vi "nufern common operation test.vi"() -> ()   [LabVIEW 2016]
uses:
  Common Operation Control 1.ctl
  Logistics Control 2.ctl
  2 digit hex indicator.ctl
  Extended Operation Control 3.ctl
  sniper current tests/Return Code Cluster.ctl
  producer enum control.ctl
  sniper current tests/Unit Status Cluster Control 1.ctl
  sniper current tests/Status  Cluster.ctl
  sniper current tests/Fault Cluster.ctl
  <vilib>/Instr/_visa.llb/VISA Configure Serial Port (Instr).vi
  <extravilib>/ChannelInstances/One Element Stream-i32/Instantiate.vi
  <extravilib>/ChannelInstances/One Element Stream-i32/EndpointRead.vi
  <extravilib>/ChannelInstances/One Element Stream-i32/Endpoint.vi
  <extravilib>/ChannelInstances/One Element Stream-i32.lvlib
panel:
  out "Fault Cluster":T1
  out "Status Cluster":T2
  out "inside Common Operation":bool
  out "Unit Status Cluster":T3={"laser serial number"=0, "Firmware Part Number"=0, "Firmware Version Major"=1, "Firmware Version Minor"=1, "Firmware Version Bugfix"=1, "Gateware Part Number"=0, "Gateware Version Minor"=1, "Gateware Version Major"=1, "Gateware Version Bugfix"=1, "Valid Readings"=FALSE} {"Gateware Version Bugfix" format="0x%02x"; "Gateware Version Major" format="0x%02x"; "Gateware Version Minor" format="0x%02x"; "Gateware Part Number" format="0x%04x"; "Firmware Version Bugfix" format="0x%02x"; "Firmware Version Minor" format="0x%02x"; "Firmware Version Major" format="0x%02x"; "Firmware Part Number" format="0x%04x"}
  out "return count 2":u32
  out "read buffer":string
  in  "control":T5=enum."Common Operation"
  out "New Value Could not be parsed":bool
  out "New value is outside \nof the inclusive range of 1-99%":bool
  out "Fault Status Cluster":T6
  out "Extended Status Cluster":T7 {"Temperature Array" format="0x%02x"; "Back-Reflection" format="0x%08x"; "HPE Threshold" format="0x%08x"; "HPE Monitor" format="0x%08x"; "Stage 2 Output Monitor" format="0x%08x"; "Stage 1 Input Monitor" format="0x%08x"; "Stage 2 Current" format="0x%08x"; "Stage 1 Current" format="0x%08x"; "Extended Status Return Code" format="0x%02x"}
  out "Back-Reflection Reading":u32 format="0x%08x"
  out "Return Code Cluster":T8 {"Current RS-485 \nAddress" format="0x%02x"; "Desired RS-485 \nAddress" format="0x%02x"; "Set Power Mode Return Code" format="0x%02x"; "Clear Faults Return Code" format="0x%02x"; "Return Code Description" items=["Accepted/No Error", "Incorrect Message Format", "Incorrect Message Length", "CRC Error", "Unrecognized Command", "Argument Out of Range", "Argument Parse Error", "Operation Not Permitted", "Operation Failed"]; "Get RS-485 Address \nReturn Code" format="0x%02x"; "Set RS-485 Address \nReturn Code" format="0x%02x"; "Set Power Mode Return Code" format="0x%02x"; "Clear Faults Return Code" format="0x%02x"; "Extended Status Return Code" format="0x%02x"}
  out "HPE Photodiode Reading":u32 format="0x%08x"
  out "Laser is in High Power Mode":bool
  out "aborted?":bool
  in  "timeout (s)":dbl=1.0 format="%#_13g"
  out "consumer loop":i32
  out "stop consumer":bool
  out "producer loop":i32
  out "stop producer":bool
  in  "stop":bool
  out "return count":u32
  out "string out to nufern":string
  in  "PAPA Address":i8=1 format="0x%02x"
  in  "Calibration":T9 {"Common Operation" format="0x%d" items=["Undefined", "Query: Get Unit Information", "Cmd: Emission On", "Cmd: Emission Off", "Query: Get Basic Status", "Query: Get Core Status", "Query: Get Extended Status", "Cmd: Clear Faults", "Cmd: Set Power Mode"]}
  in  "Extended Operation":T10={"Extended Operation"=0, "OK Button"=FALSE, " HPE Photodiode \nSignal Drop Tolerance"=0.99} {"HPE Photodiode \nSignal Drop Tolerance" min=0.01 max=0.99 step=0.01 format="%#_g%%"; "Extended Operation" format="0x%x" items=["undefined"=0, "Set HPE Photodiode Signal Drop Tolerance"=67, "Get HPE Photodiode Signal Drop Tolerance"=68, "Switch HPE Photodiode Fault Enable"=69, "Get Temperature Sensor Status"=70, "Switch Communication Timeout Enable"=71]}
  in  "Logistics":T11={"Logistics"=66, "OK Button"=FALSE, "Desired RS-485 \nAddress "=0, "Current RS-485 \nAddress "=0} {"Current RS-485 \nAddress" format="0x%02x"; "Desired RS-485 \nAddress" format="0x%02x"; "Logistics" format="0x%x" items=["Set RS-485 Address"=65, "Get RS-485 Address"=66]}
  in  "Common Operation":T9={"Common Operation"=1, "OK Button"=FALSE} {"Common Operation" format="0x%d" items=["Undefined", "Query: Get Unit Information", "Cmd: Emission On", "Cmd: Emission Off", "Query: Get Basic Status", "Query: Get Core Status", "Query: Get Extended Status", "Cmd: Clear Faults", "Cmd: Set Power Mode"]}
  out "error out":errorcluster
  in  "error in (no error)":errorcluster
  in  "baud rate (9600)":u32=115200
  in  "VISA resource name":refnum<visa-resource-name>="COM1"
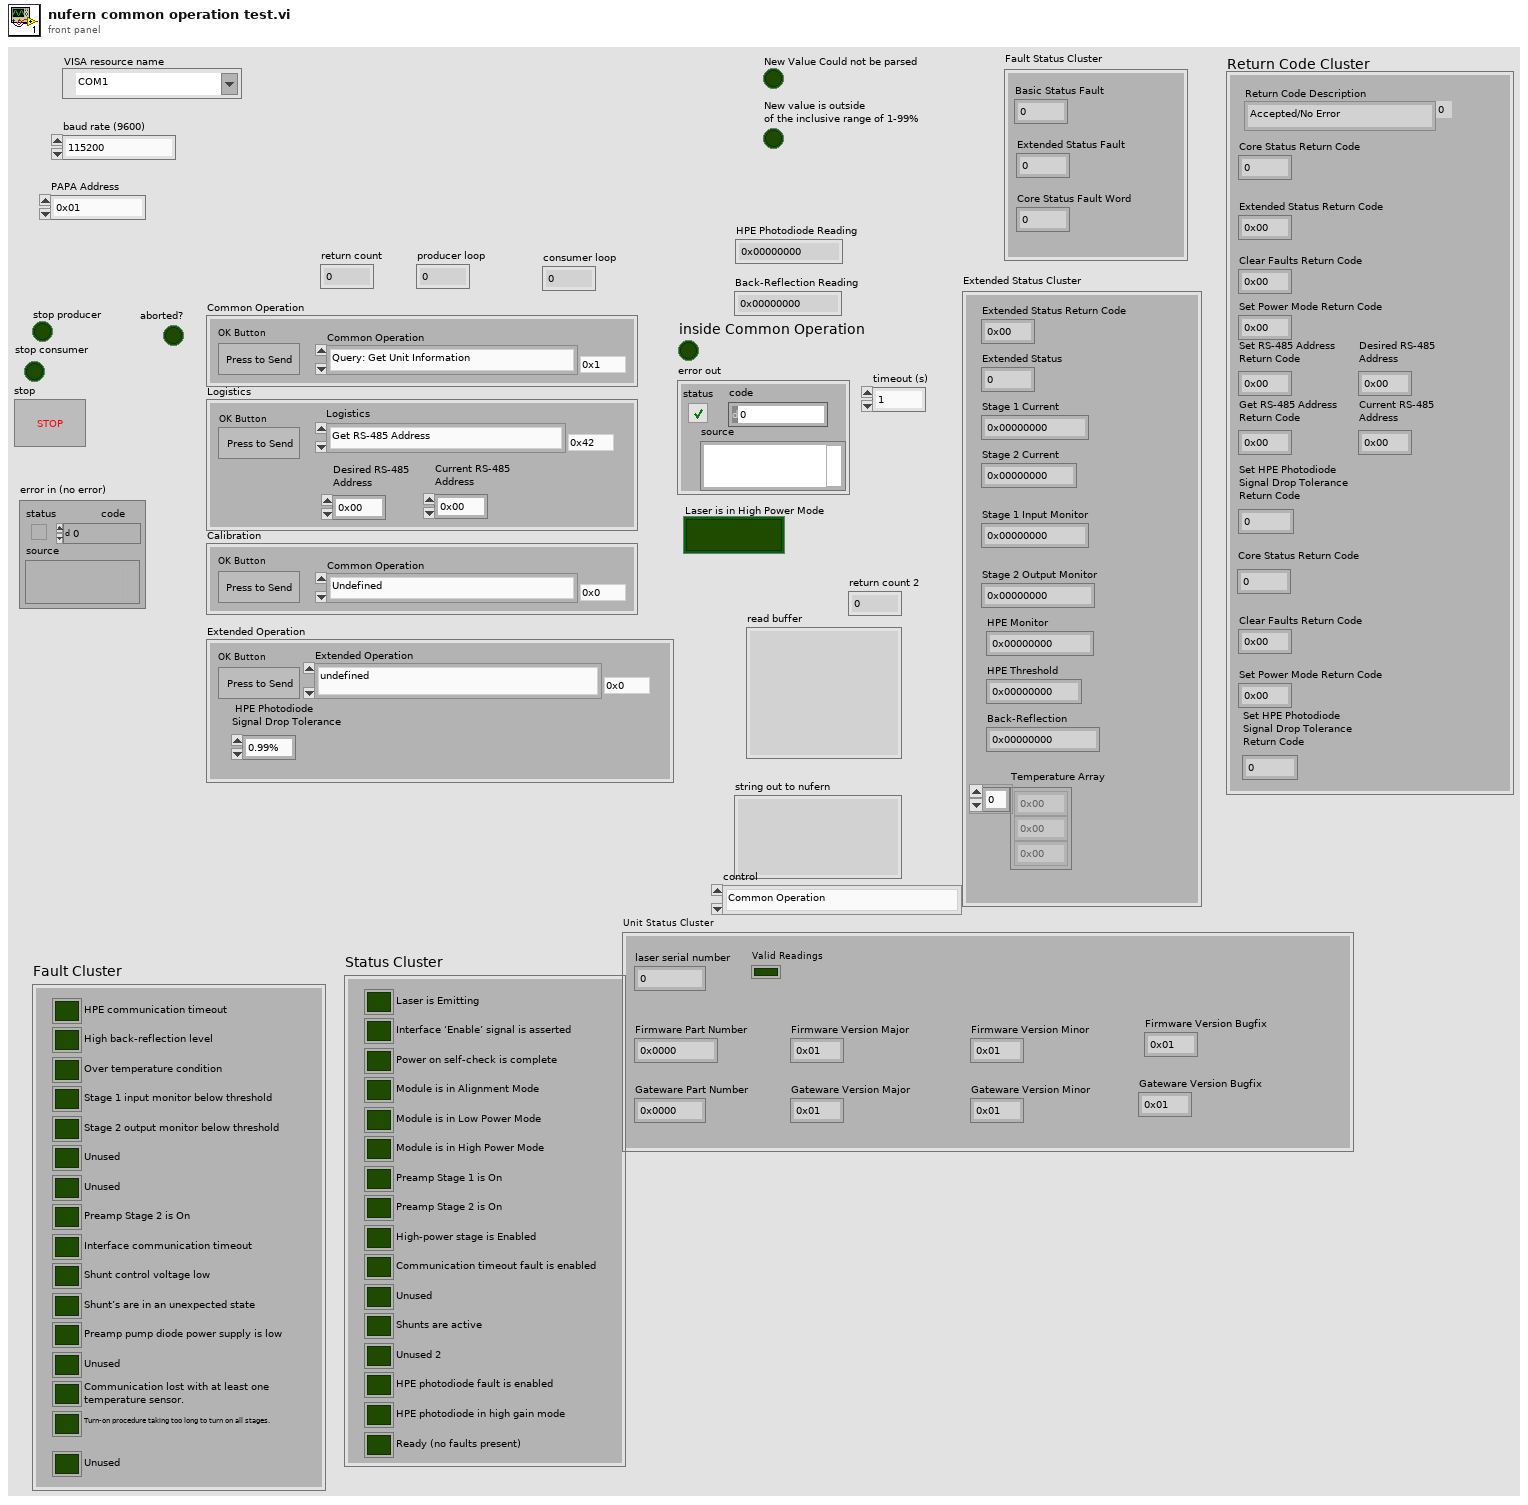
[diagram p1: front panel]
types:
  T1 = typedef "Fault Cluster.ctl" = cluster{"HPE communication timeout":bool, "High back-reflection level":bool, "Over temperature condition":bool, "Stage 1 input monitor below threshold":bool, "Stage 2 output monitor below threshold":bool, "Unused":bool, "Unused":bool, "Preamp Stage 2 is On":bool, "Interface communication timeout":bool, "Shunt control voltage low":bool, "Shunt’s are in an unexpected state":bool, "Preamp pump diode power supply is low":bool, "Unused":bool, "Communication lost with at least one\ntemperature sensor.":bool, "Turn-on procedure taking too long to turn on all stages.":bool, "Unused":bool}
  T2 = typedef "Status  Cluster.ctl" = cluster{"Laser is Emitting":bool, "Interface ‘Enable’ signal is asserted":bool, "Power on self-check is complete":bool, "Module is in Alignment Mode":bool, "Module is in Low Power Mode":bool, "Module is in High Power Mode":bool, "Preamp Stage 1 is On":bool, "Preamp Stage 2 is On":bool, "High-power stage is Enabled":bool, "Communication timeout fault is enabled":bool, "Unused":bool, "Shunts are active":bool, "Unused 2":bool, "HPE photodiode fault is enabled":bool, "HPE photodiode in high gain mode":bool, "Ready (no faults present)":bool}
  T3 = typedef "Unit Status Cluster Control 1.ctl" = cluster{"laser serial number":u32, "Firmware Part Number":u32, "Firmware Version Major":T4, "Firmware Version Minor":T4, "Firmware Version Bugfix":T4, "Gateware Part Number":u32, "Gateware Version Minor":T4, "Gateware Version Major":T4, "Gateware Version Bugfix":T4, "Valid Readings":bool}
  T4 = typedef "2 digit hex indicator.ctl" = i32
  T5 = typedef "producer enum control.ctl" = enum16{"Timeout", "Stop", "Common Operation", "Calibration", "Extended Operation", "Logistics"}
  T6 = cluster{"Basic Status Fault":u32, "Core Status Fault Word":u32, "Extended Status Fault":u32}
  T7 = cluster{"Extended Status Return Code":T4, "Extended Status ":u32, "Stage 1 Current":u32, "Stage 2 Current":u32, "Stage 1 Input Monitor":u32, "Stage 2 Output Monitor":u32, "HPE Monitor":u32, "HPE Threshold":u32, "Back-Reflection":u32, "Temperature Array":T4[]}
  T8 = typedef "Return Code Cluster.ctl" = cluster{"Core Status Return Code":u32, "Extended Status Return Code":T4, "Clear Faults Return Code":T4, "Set Power Mode Return Code":T4, "Set RS-485 Address \nReturn Code":T4, "Get RS-485 Address \nReturn Code":T4, "Set HPE Photodiode \nSignal Drop Tolerance \nReturn Code":u32, "Return Code Description":u16, "Core Status Return Code":u32, "Clear Faults Return Code":T4, "Set Power Mode Return Code ":T4, "Desired RS-485 \nAddress ":T4, "Current RS-485 \nAddress ":T4, "Set HPE Photodiode \nSignal Drop Tolerance \nReturn Code ":u32}
  T9 = typedef "Common Operation Control 1.ctl" = cluster{"Common Operation":u16, "OK Button":bool}
  T10 = typedef "Extended Operation Control 3.ctl" = cluster{"Extended Operation":u16, "OK Button":bool, " HPE Photodiode \nSignal Drop Tolerance":dbl}
  T11 = typedef "Logistics Control 2.ctl" = cluster{"Logistics":u16, "OK Button":bool, "Desired RS-485 \nAddress ":T4, "Current RS-485 \nAddress ":T4}
  T12 = typedef "One Element Stream-i32.lvlib/)Channel.ctl" = refnum<queue>
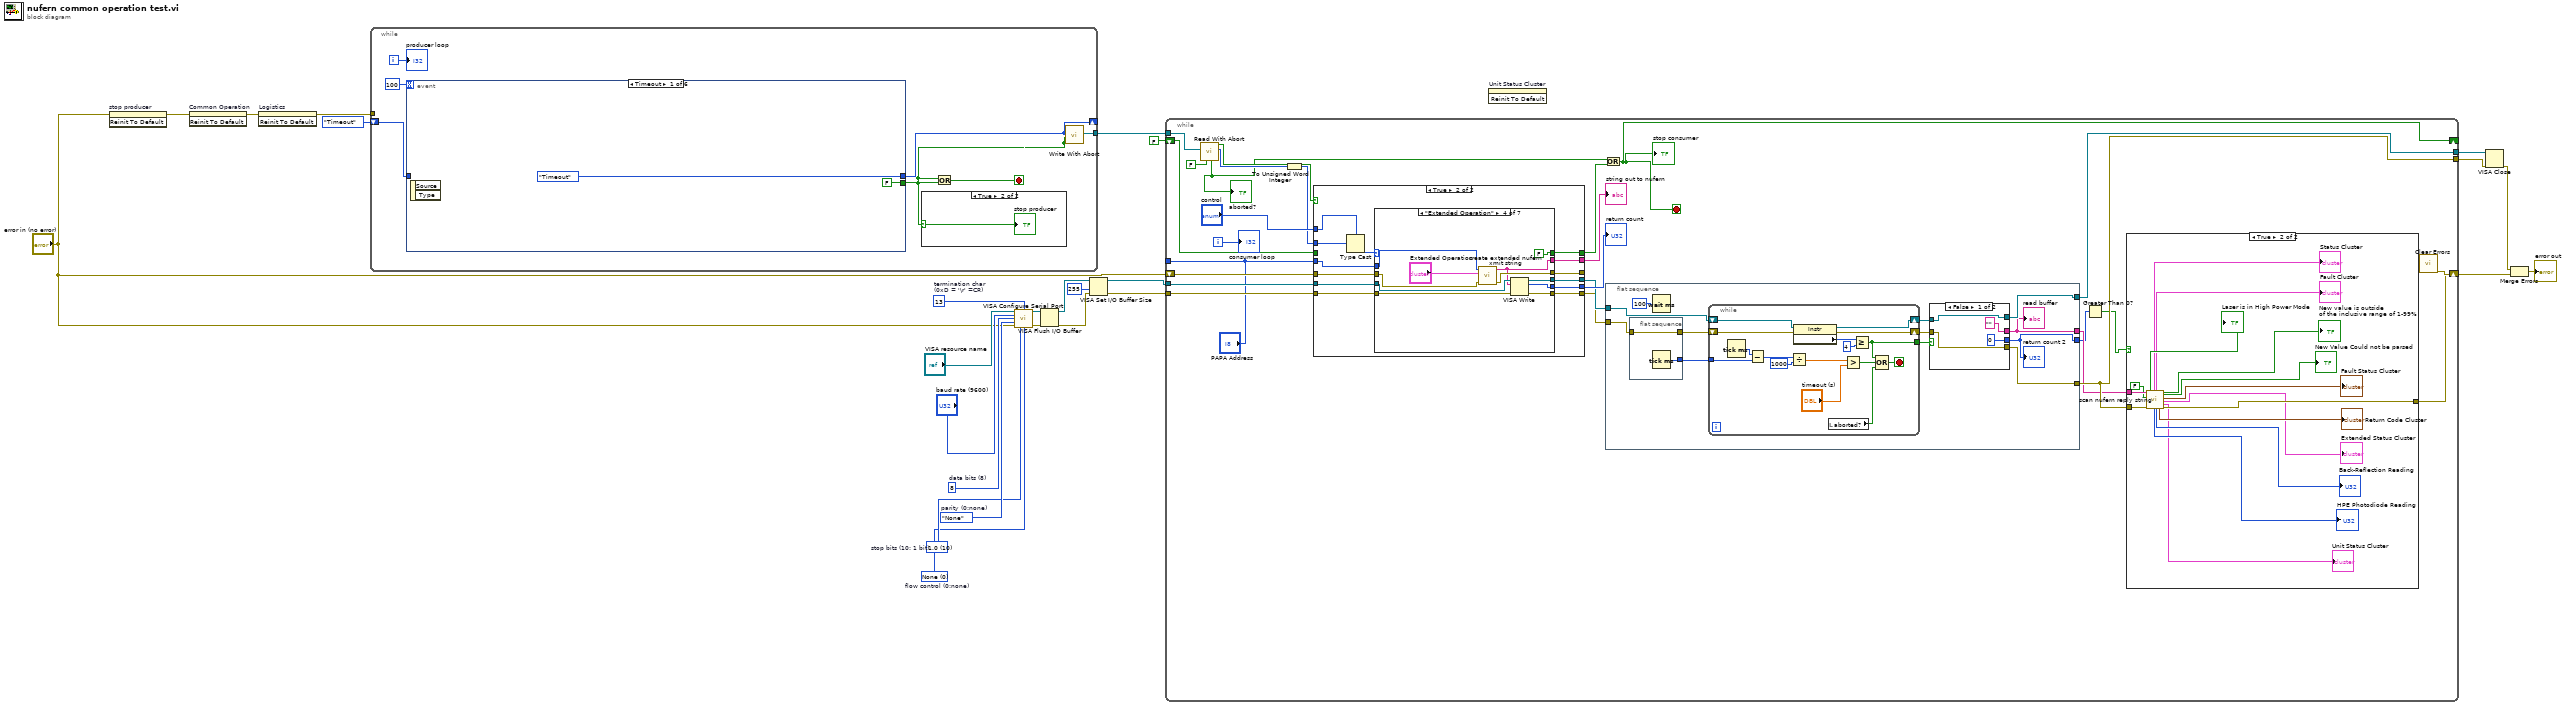
[diagram p0: block diagram]
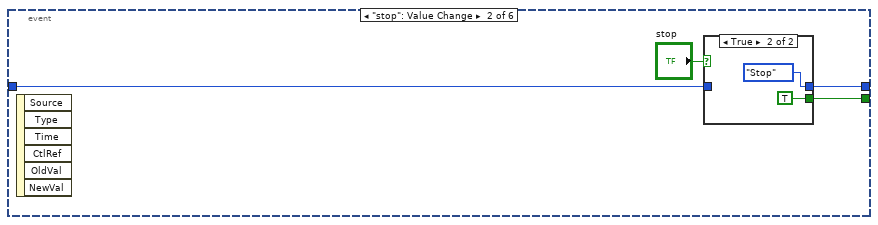
[diagram p2: hidden frame]
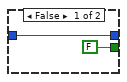
[diagram p3: hidden frame]
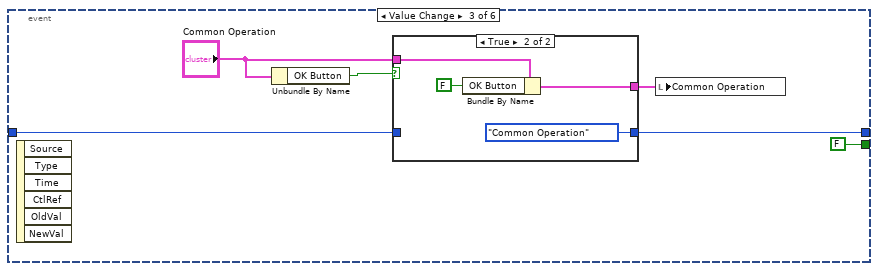
[diagram p4: hidden frame]
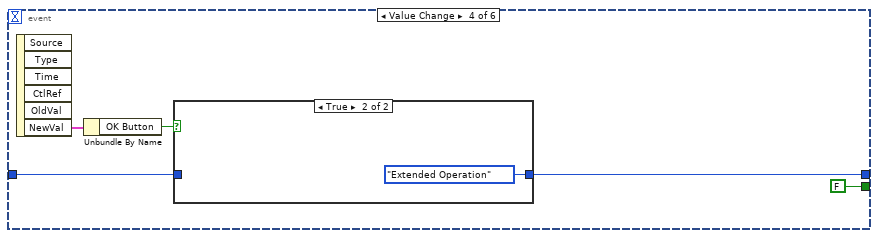
[diagram p6: hidden frame]
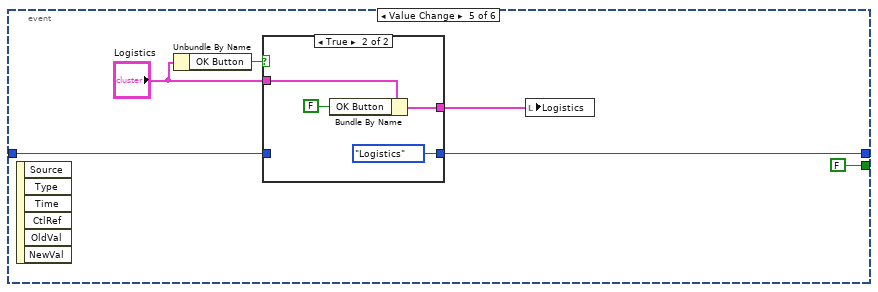
[diagram p8: hidden frame]
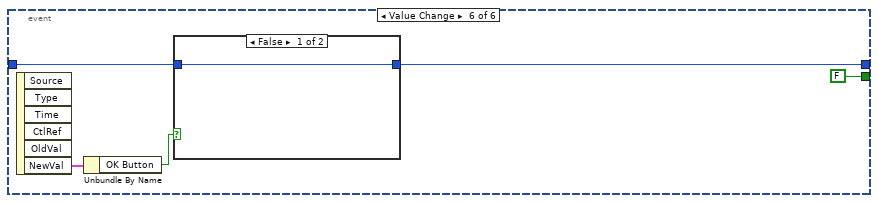
[diagram p10: hidden frame]
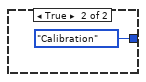
[diagram p11: hidden frame]
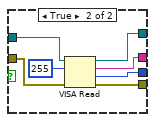
[diagram p14: hidden frame]
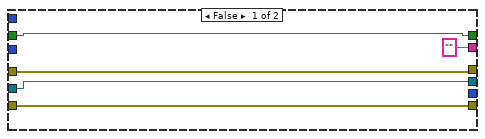
[diagram p15: hidden frame]
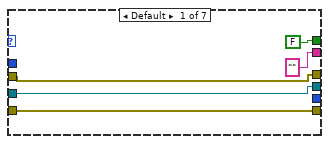
[diagram p16: hidden frame]
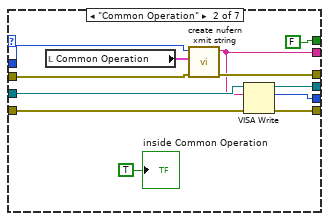
[diagram p17: hidden frame]
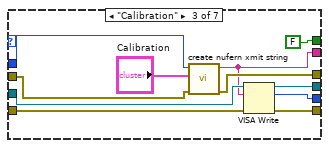
[diagram p18: hidden frame]
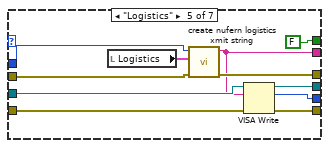
[diagram p19: hidden frame]
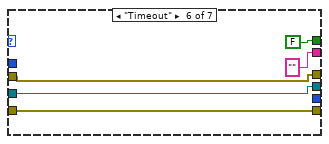
[diagram p20: hidden frame]
diagram:
  w18 = u8 13  # termination char (0xD = '\r' =CR)
  w21 = u16 0 items=["None", "XON/XOFF", "RTS/CTS", "XON/XOFF & RTS/CTS", "DTR/DSR", "XON/XOFF & DTR/DSR"]  # flow control (0:none)
  w22 = u16 10 items=["1.0"=10, "1.5"=15, "2.0"=20]  # stop bits (10: 1 bit)
  w23 = enum16{"None", "Odd", "Even", "Mark", "Space"}."None"  # parity (0:none)
  w24 = u16 8  # data bits (8)
  n1 = invoke on="stop producer" class="Bool (strict)" method="Reinit To Default"(error in="error in (no error)") -> (error out=w1:errorcluster)  [unwired: 2 in, 2 out]
  n2 = invoke on="Common Operation" class="Clust (strict)" method="Reinit To Default"(error in=w1) -> (error out=w4:errorcluster)  [unwired: 2 in, 2 out]
  n3 = invoke on="Logistics" class="Clust (strict)" method="Reinit To Default"(error in=w4) -> (error out=w3:errorcluster)  [unwired: 2 in, 2 out]
  n4 = while {
    tunnel: [w31] -> w12
    shift-right: [w28] -> _
    shift-left: producer_enum_control."Timeout" -> [w29]
    tunnel: w3 -> [_]
    i -> [w32]
    stop <- w30 stop-if-true
    n5 = event shown="[0] Timeout" {
      selector: _ -> [_ _ _ _ _ _]
      dyn-events: _ -> [_ _ _ _ _ _]
      timeout: 100 -> [_ _ _ _ _ _]
      tunnel: [producer_enum_control."Timeout" w38 w49 w60 w68 w79] -> w28
      tunnel: w29 -> [_ w36 w47 w57 w66 w76]
      tunnel: [FALSE w37 FALSE FALSE FALSE FALSE] -> w27
      event Timeout {
        n6 = event-data() -> ()  [unwired: 1 in, 2 out]
      }
      event "stop": Value Change {
        n7 = event-data() -> ()  [unwired: 1 in, 6 out]
        n8 = case shown="True" "stop" {
          tunnel: [w40 producer_enum_control."Stop"] -> w38
          tunnel: [FALSE TRUE] -> w37
          tunnel: w36 -> [w40 _]
          frame False {
          }
          frame True {
          }
        }
      }
      event Value Change {
        n9 = event-data() -> ()  [unwired: 1 in, 6 out]
        n10 = Unbundle By Name("Common Operation") -> ("OK Button"=w46:bool)
        n11 = case shown="True" w46 {
          tunnel: [w51 producer_enum_control."Common Operation"] -> w49
          tunnel: w47 -> [w51 _]
          tunnel: [w50 w53] -> w45
          tunnel: "Common Operation" -> [w50 w54]
          frame False {
          }
          frame True {
            n12 = Bundle By Name(cluster=w54, "OK Button"=FALSE) -> (w53:T9)
          }
        }
        n13 = local write "Common Operation"(w45) -> ()
      }
      event Value Change {
        n14 = event-data() -> ("NewVal"=w58:T10)  [unwired: 1 in, 5 out]
        n15 = Unbundle By Name(w58) -> ("OK Button"=w56:bool)
        n16 = case shown="True" w56 {
          tunnel: [w61 producer_enum_control."Extended Operation"] -> w60
          tunnel: w57 -> [w61 _]
          frame False {
          }
          frame True {
          }
        }
      }
      event Value Change {
        n17 = event-data() -> ()  [unwired: 1 in, 6 out]
        n18 = Unbundle By Name("Logistics") -> ("OK Button"=w65:bool)
        n19 = case shown="True" w65 {
          tunnel: [w70 producer_enum_control."Logistics"] -> w68
          tunnel: w66 -> [w70 _]
          tunnel: [w69 w72] -> w64
          tunnel: "Logistics" -> [w69 w73]
          frame False {
          }
          frame True {
            n20 = Bundle By Name(cluster=w73, "OK Button"=FALSE) -> (w72:T11)
          }
        }
        n21 = local write "Logistics"(w64) -> ()
      }
      event Value Change {
        n22 = event-data() -> ("NewVal"=w77:T9)  [unwired: 1 in, 5 out]
        n23 = Unbundle By Name(w77) -> ("OK Button"=w75:bool)
        n24 = case shown="False" w75 {
          tunnel: [w80 producer_enum_control."Calibration"] -> w79
          tunnel: w76 -> [w80 _]
          frame False {
          }
          frame True {
          }
        }
      }
    }
    n25 = case shown="True" w27 {
      selector: w27 -> [_ w82]
      frame False {
      }
      frame True {
        "stop producer" <- w82
      }
    }
    n26 = Or(x=w27, y=w27) -> (x .or. y?=w30:bool)
    n27 = call <extravilib>:"Write With Abort.vi"("abort"=w27, "last element? (F)"=w27, "element"=w28) -> ("channel"=w31:T12)  [unwired: 6 in, 2 out]
    "producer loop" <- w32
  }
  n28 = call-poly "VISA Configure Serial Port"("VISA resource name"="VISA resource name", "termination char\n(0xA = '\\n' = LF)"=w18, "baud rate (9600)"="baud rate (9600)", "data bits (8)"=w24, "parity (0:none)"=w23, "error in (no error)"="error in (no error)", "stop bits (10: 1 bit)"=w22, "flow control (0:none)"=w21) -> ("VISA resource name out"=w19:refnum<visa-resource-name>, "error out"=w20:errorcluster)  [unwired: 6 in]
  n29 = VISA Flush I/O Buffer(VISA resource name=w19, error in (no error)=w20) -> (VISA resource name out=w15:refnum<visa-resource-name>, error out=w7:errorcluster)  [unwired: 1 in]
  n30 = VISA Set I/O Buffer Size(VISA resource name=w15, size (4096)=u32 255, error in (no error)=w7) -> (VISA resource name out=w8:refnum<visa-resource-name>, error out=w6:errorcluster)  [unwired: 1 in]
  n31 = while {
    shift-right: [w93] -> w9
    shift-left: "error in (no error)" -> [w108]
    tunnel: w8 -> [w107]
    tunnel: [w91] -> w14
    tunnel: w6 -> [w106]
    tunnel: [w90] -> w13
    tunnel: ["PAPA Address"] -> _
    tunnel: w12 -> [w104]
    shift-right: [w95] -> _
    shift-left: FALSE -> [w98]
    i -> [w100]
    stop <- w95 stop-if-true
    n32 = call <extravilib>:"Read With Abort.vi"("abort"=FALSE, "channel"=w104) -> ("element"=w102:i32, "element valid?"=w103:bool, "aborted?"=w94:bool)  [unwired: 5 in, 2 out]
    "aborted?" <- w94
    n33 = To Unsigned Word Integer(number=w102) -> (unsigned 16bit integer=w85:u16)
    n34 = case shown="True" w103 {
      tunnel: [w168 w183] -> _
      tunnel: w108 -> [w168 w182]
      tunnel: w107 -> [w170 w181]
      tunnel: "PAPA Address" -> [_ w180]
      tunnel: [w170 w179] -> w97
      tunnel: w106 -> [w169 w178]
      tunnel: [w169 w177] -> w96
      tunnel: ["" ("String Out to nufern") w176] -> w89
      tunnel: [_ w175] -> w105
      tunnel: "control" -> [_ w173]
      tunnel: w85 -> [_ w171]
      tunnel: [w166 w174] -> w99
      tunnel: w98 -> [w166 _]
      frame False {
      }
      frame True {
        n35 = Type Cast(type=w173, x=w171) -> (*(type *) &x=w172:T5)
        n36 = case shown="\"Extended Operation\"" w172 {
          tunnel: [w186 w200 w211 w222 w233 w237 w241] -> w183
          tunnel: w182 -> [w186 w199 w210 w221 w232 w237 w241]
          tunnel: w181 -> [w188 w198 w209 w220 w231 w235 w239]
          tunnel: w180 -> [_ w197 w208 w219 w230 _ _]
          tunnel: [w188 w196 w207 w218 w229 w235 w239] -> w179
          tunnel: w178 -> [w187 w195 w206 w217 w228 w236 w240]
          tunnel: [w187 w194 w205 w216 w227 w236 w240] -> w177
          tunnel: ["" ("String Out to nufern") w191 w204 w215 w226 "" ("String Out to nufern") _] -> w176
          tunnel: [_ w193 w203 w214 w225 _ _] -> w175
          tunnel: [FALSE FALSE FALSE FALSE FALSE FALSE TRUE] -> w174
          frame Default {
          }
          frame "Common Operation" {
            n37 = local read "Common Operation"() -> (w190:T9)
            n38 = call "create nufern xmit string.vi"("error in (no error)"=w199, "Common Operation"=w190, "PAPA Address"=w197) -> ("error out"=w200:errorcluster, "String Out to nufern"=w191:string)  [unwired: 5 in, 2 out]
            n39 = VISA Write(VISA resource name=w198, write buffer=w191, error in (no error)=w195) -> (VISA resource name out=w196:refnum<visa-resource-name>, return count=w193:u32, error out=w194:errorcluster)
            "inside Common Operation" <- TRUE
          }
          frame "Calibration" {
            n40 = call "create nufern xmit string.vi"("error in (no error)"=w210, "Common Operation"="Calibration", "PAPA Address"=w208) -> ("error out"=w211:errorcluster, "String Out to nufern"=w204:string)  [unwired: 5 in, 2 out]
            n41 = VISA Write(VISA resource name=w209, write buffer=w204, error in (no error)=w206) -> (VISA resource name out=w207:refnum<visa-resource-name>, return count=w203:u32, error out=w205:errorcluster)
          }
          frame "Extended Operation" {
            n42 = call "create extended nufern xmit string.vi"("error in (no error)"=w221, "Extended Operation"="Extended Operation", "PAPA Address"=w219) -> ("error out"=w222:errorcluster, "String Out to nufern"=w215:string)  [unwired: 5 in, 2 out]
            n43 = VISA Write(VISA resource name=w220, write buffer=w215, error in (no error)=w217) -> (VISA resource name out=w218:refnum<visa-resource-name>, return count=w214:u32, error out=w216:errorcluster)
          }
          frame "Logistics" {
            n44 = local read "Logistics"() -> (w223:T11)
            n45 = call "create nufern logistics xmit string.vi"("error in (no error)"=w232, "Logistics Operation"=w223, "PAPA Address"=w230) -> ("error out"=w233:errorcluster, "String Out to nufern"=w226:string)  [unwired: 5 in, 2 out]
            n46 = VISA Write(VISA resource name=w231, write buffer=w226, error in (no error)=w228) -> (VISA resource name out=w229:refnum<visa-resource-name>, return count=w225:u32, error out=w227:errorcluster)
          }
          frame "Timeout" {
          }
          frame "Stop" {
          }
        }
      }
    }
    "return count" <- w105
    "string out to nufern" <- w89
    n47 = Or(x=w94, y=w99) -> (x .or. y?=w95:bool)
    "stop consumer" <- w95
    n48 = flat-sequence {
      tunnel: w97 -> [w136]
      tunnel: w96 -> [w135]
      tunnel: [w129] -> w91
      tunnel: [w128] -> w90
      tunnel: [w126] -> w88
      tunnel: [w125] -> w87
      frame #0 {
        n49 = flat-sequence {
          tunnel: w135 -> [w138]
          tunnel: [w138] -> w134
          tunnel: [w137] -> w133
          frame #0 {
            n50 = Tick Count (ms)() -> (millisecond timer value=w137:u32)
          }
        }
        n51 = Wait (ms)(milliseconds to wait=u32 100) -> ()  [unwired: 1 out]
        n52 = while {
          shift-right: [w164] -> w130
          shift-left: w134 -> [w165]
          shift-right: [w162] -> w132
          shift-left: w136 -> [w163]
          tunnel: w133 -> [w159]
          tunnel: [w152] -> w131
          stop <- w154 stop-if-true
          n53 = Tick Count (ms)() -> (millisecond timer value=w160:u32)
          n54 = Subtract(x=w160, y=w159) -> (x-y=w158:u32)
          n55 = Divide(x=w158, y=u32 1000) -> (x/y=w156:dbl)
          n56 = property class="Instr"(reference=w163, error in=w165) -> (reference out=w162:refnum<visa-resource-name>, error out=w164:errorcluster, "Serial Settings:Number of Bytes at Serial Port"=w151:u32)
          n57 = local read "aborted?"() -> (w150:bool)
          n58 = Greater?(x=w156, y="timeout (s)") -> (0:w153:bool)
          n59 = Greater Or Equal?(x=w151, y=u32 4) -> (x >= y?=w152:bool)
          n60 = Compound Arithmetic op=OR(w152, w153, w150) -> (w154:bool)
        }
        n61 = case shown="False" w131 {
          tunnel: w132 -> [w142 w149]
          tunnel: [w142 w148] -> w129
          tunnel: w130 -> [w141 w147]
          tunnel: [w141 w145] -> w128
          tunnel: ["" ("read buffer") w144] -> w126
          tunnel: [u32 0 ("return count") w143] -> w125
          frame False {
          }
          frame True {
            n62 = VISA Read(VISA resource name=w149, byte count=u32 255, error in (no error)=w147) -> (VISA resource name out=w148:refnum<visa-resource-name>, read buffer=w144:string, return count=w143:u32, error out=w145:errorcluster)
          }
        }
        "read buffer" <- w126
        "return count 2" <- w125
      }
    }
    n63 = Greater Than 0?(x=w87) -> (x > 0?=w83:bool)
    n64 = case shown="True" w83 {
      tunnel: [w109 w124] -> w92
      tunnel: w90 -> [w109 w123]
      tunnel: w88 -> [_ w122]
      frame False {
      }
      frame True {
        n65 = call "scan nufern reply string.vi"("Input String"=w122, "Manual"=FALSE, "error in (no error)"=w123) -> ("Laser is in High Power Mode"=→"Laser is in High Power Mode":bool, "Status Cluster"=→"Status Cluster":T2, "HPE Photodiode Reading"=→"HPE Photodiode Reading":u32, "Fault Cluster"=→"Fault Cluster":T1, "Back-Reflection Reading"=→"Back-Reflection Reading":u32, "Return Code Cluster"=→"Return Code Cluster":T8, "New value is outside \nof the inclusive range of 1-99%"=→"New value is outside \nof the inclusive range of 1-99%":bool, "New Value Could not be parsed"=→"New Value Could not be parsed":bool, "Fault Status Cluster"=→"Fault Status Cluster":T6, "Extended Status Cluster"=→"Extended Status Cluster":T7, "Unit Status Cluster"=→"Unit Status Cluster":T3, "error out"=w124:errorcluster)  [unwired: 5 in]
      }
    }
    n66 = call <vilib>:"Clear Errors.vi"("error in (no error)"=w92) -> ("error out"=w93:errorcluster)  [unwired: 5 in, 1 out]
    "consumer loop" <- w100
  }
  n67 = invoke on="Unit Status Cluster" class="Clust (strict)" method="Reinit To Default"() -> ()  [unwired: 3 in, 3 out]
  n68 = VISA Close(VISA resource name=w14, error in (no error)=w13) -> (error out=w16:errorcluster)
  n69 = Merge Errors(w16, w9) -> (→"error out":errorcluster)
